vi "Poly Eigenvectors from Input Matrices Eigenvalues and Vectors (DBL).vi"(9 "Eigenvectors":T1, 10 "Eigenvalues":cdb[](array[numeric]), 11 "Input Matrices":dbl[][][](array[numeric])) -> (3 "X":T1)   [LabVIEW 2010, in "NI_AALPro.lvlib"]
uses:
  NI_AALPro.lvlib
  ComplexMatrix.ctl
  Complex A x B.vi
  NI_AALBase.lvlib
  NI_Matrix.lvlib
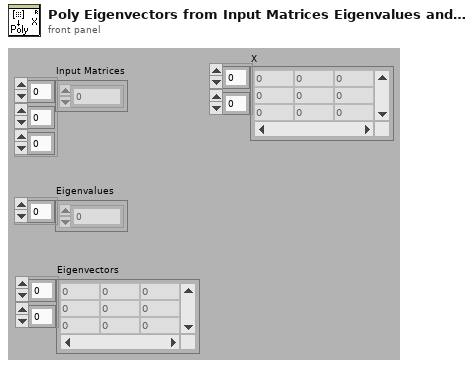
[diagram p1: front panel]
types:
  T1 = typedef "NI_Matrix.lvlib/ComplexMatrix.ctl" = cdb[][]
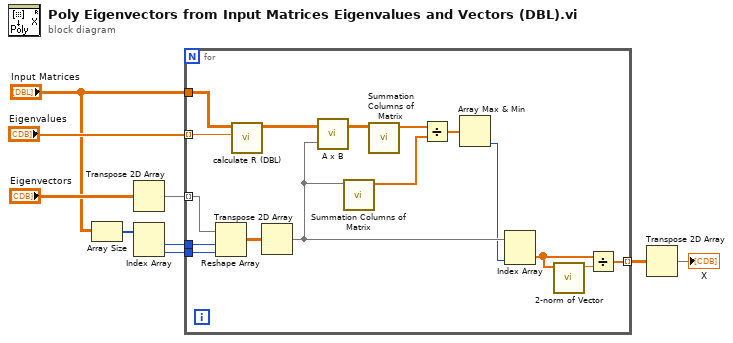
[diagram p0: block diagram]
diagram:
  n1 = Array Size(array="Input Matrices") -> (size(s)=w3:i32[])
  n2 = Transpose 2D Array(2D array="Eigenvectors") -> (transposed array=w8:T1)
  n3 = Index Array(array=w3) -> (element #1=w2:i32, element #2=w1:i32)  [unwired: 2 in]
  n4 = for {
    tunnel: w8 -> [w25] mode=indexing
    tunnel: w2 -> [w24]
    tunnel: w1 -> [w23]
    tunnel: "Eigenvalues" -> [w21] mode=indexing
    tunnel: "Input Matrices" -> [w20]
    tunnel: [w10] -> w6 mode=indexing
    n5 = Reshape Array(w25, w24, w23) -> (w22:cdb[][])
    n6 = call "calculate R (DBL).vi"("eigenvalue"=w21, "Array"=w20) -> ("R"=w19:cdb[][])  [unwired: 9 in]
    n7 = Transpose 2D Array(2D array=w22) -> (transposed array=w14:cdb[][])
    n8 = call-poly "A x B.vi"("B"=w14, "A"=w19) -> ("A x B"=w18:T1)  [unwired: 1 out]
    n9 = call "Summation Columns of Matrix.vi"("A"=w14) -> ("Summation Columns of A"=w16:dbl[])  [unwired: 10 in]
    n10 = call "Summation Columns of Matrix.vi"("A"=w18) -> ("Summation Columns of A"=w17:dbl[])  [unwired: 10 in]
    n11 = Divide(x=w17, y=w16) -> (x/y=w15:dbl[])
    n12 = Array Max & Min(array=w15) -> (min index (indices)=w13:i32)  [unwired: 3 out]
    n13 = Index Array(array=w14, index (col)=w13) -> (element=w11:cdb[])  [unwired: 1 in]
    n14 = call "2-norm of Vector.vi"("V"=w11) -> ("2-norm of V"=w12:dbl)  [unwired: 10 in]
    n15 = Divide(x=w11, y=w12) -> (x/y=w10:cdb[])
  }
  n16 = Transpose 2D Array(2D array=w6) -> (transposed array=→"X":cdb[][])
